vi "Windows Title.vi"(8 "error in (no error)":errorcluster, 9 "Data":string, 10 "ActorQName":string, 11 "CallActorCenter in":refnum<class "CallActorCenter.lvclass">) -> (0 "error out":errorcluster, 3 "CallActorCenter out":refnum<class "CallActorCenter.lvclass">)   [LabVIEW 2021, in "CallActorCenter.lvclass"]
uses:
  CallActorCenter.lvclass
  CallActorCenter.lvclass/CallActorCenter.ctl
  <userlib>/John_Lib/AbstractActorTemplate/AbstractActorTemplate/UIActorTop.lvclass
  <userlib>/John_Lib/Interfaces/Windows Title Messages/Windows Title Msg/Windows Title Msg.lvclass
  C:/Program Files (x86)/National Instruments/LabVIEW 2021/user.lib/John_Lib/AbstractActorTemplate/AbstractActorTemplate/UIActorTop.lvclass
  C:/Program Files (x86)/National Instruments/LabVIEW 2021/vi.lib/ActorFramework/Actor/Actor.lvclass
  C:/Program Files (x86)/National Instruments/LabVIEW 2021/project/Create Actor from Template/_CallActorCenter/CallActorCenter.lvclass
  C:/Program Files (x86)/National Instruments/LabVIEW 2021/user.lib/John_Lib/Interfaces/CheckPassWord/CheckPassWord.lvclass
  C:/Program Files (x86)/National Instruments/LabVIEW 2021/user.lib/John_Lib/Interfaces/FrontPanel Save Image/FrontPanel Save Image.lvclass
  C:/Program Files (x86)/National Instruments/LabVIEW 2021/user.lib/John_Lib/Interfaces/InsertButtonSubPanel/InsertButtonSubPanel.lvclass
  C:/Program Files (x86)/National Instruments/LabVIEW 2021/user.lib/John_Lib/Interfaces/InsertLeftSubPanel/InsertLeftSubPanel.lvclass
  C:/Program Files (x86)/National Instruments/LabVIEW 2021/user.lib/John_Lib/Interfaces/InsertMainSubPanel/InsertMainSubPanel.lvclass
  C:/Program Files (x86)/National Instruments/LabVIEW 2021/user.lib/John_Lib/Interfaces/InsertRightSubPanel/InsertRightSubPanel.lvclass
  C:/Program Files (x86)/National Instruments/LabVIEW 2021/user.lib/John_Lib/Interfaces/InsertSubPanel/InsertSubPanel.lvclass
  C:/Program Files (x86)/National Instruments/LabVIEW 2021/user.lib/John_Lib/Interfaces/Windows Title/Windows Title.lvclass
  <vilib>/ActorFramework/Actor/Actor.lvclass
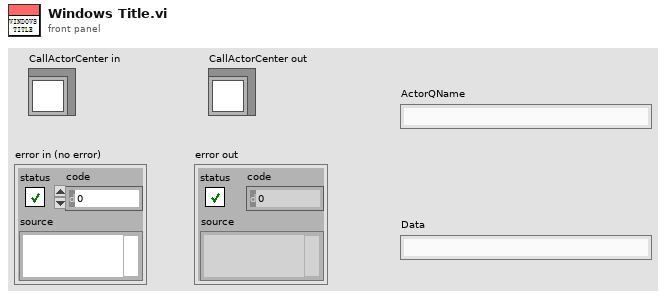
[diagram p1: front panel]
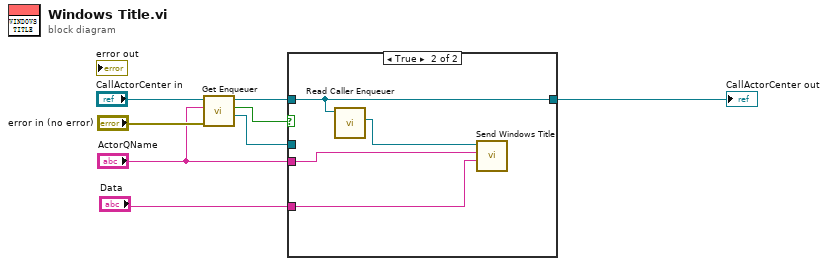
[diagram p0: block diagram]
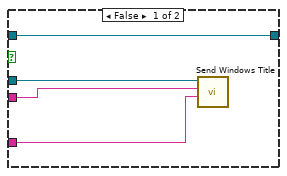
[diagram p2: hidden frame]
diagram:
  n1 = call <userlib>:"Get Enqueuer.vi"("error in (no error)"="error in (no error)", "ActorQName"="ActorQName", "UIActorTop in"="CallActorCenter in") -> ("Nested Actor's Enqueuer"=w3:refnum<class "Message Enqueuer.lvclass">, "key not found?"=w6:bool, "UIActorTop out"=w4:refnum<class "CallActorCenter.lvclass">)  [unwired: 5 in, 1 out]
  n2 = case shown="True" w6 {
    tunnel: [w12 w14] -> w5
    tunnel: w4 -> [w12 w14]
    tunnel: w3 -> [w11 _]
    tunnel: "ActorQName" -> [w10 w16]
    tunnel: "Data" -> [w9 w15]
    frame False {
      n3 = call <userlib>:"Send Windows Title.vi"("Data"=w9, "ActorQName"=w10, "Message Enqueuer"=w11) -> ()  [unwired: 7 in, 2 out]
    }
    frame True {
      n4 = call <vilib>:"Read Caller Enqueuer.vi"("Actor"=w14) -> ("Caller Enqueuer"=w13:refnum<class "Message Enqueuer.lvclass">)  [unwired: 10 in]
      n5 = call <userlib>:"Send Windows Title.vi"("Data"=w15, "ActorQName"=w16, "Message Enqueuer"=w13) -> ()  [unwired: 7 in, 2 out]
    }
  }
  "CallActorCenter out" <- w5
